vi "AddModule_Item_OnPopupMenu.vi"(11 "Object":T1) -> ()   [LabVIEW 2012]
doc: "OnPopupMenu\n\n\nInputs:\n---------------------\n- Object : U64; \n\nOutputs:\n---------------------\n\n\n----------------------------------------------\n6/8/2018 jcm\nZühlke Engineering AG\nCH-8952 Schlieren\nwww.zuehlke.com"
uses:
  <resource>/Framework/Providers/API/mxLvMenuItem.ctl
  <vilib>/Utility/config.llb/NI_LVConfig.lvlib
  <vilib>/Utility/config.llb/Read Key (String).vi
  <resource>/Framework/Providers/API/ItemRef.ctl
panel:
  out "error out":errorcluster
  in  "error in":errorcluster
  # "Connector Pane"
  # "Locals"
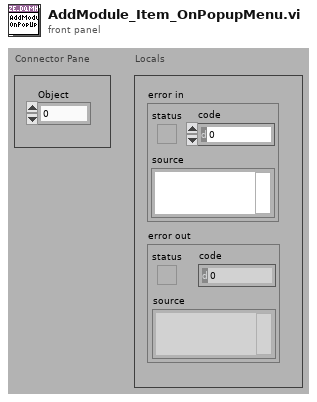
[diagram p1: front panel]
types:
  T1 = typedef "ItemRef.ctl" = u64
  T2 = typedef "mxLvMenuItem.ctl" = cluster{"Menu Name":string, "Description":string, "Icon File Name":path, "Menu Tag":string, "Enabled":bool, "Checked":bool, "Separator":bool, "Batchable":bool, "Weight":i32, "Batch Mode (Ignored if Not Batchable)":enum32{"Show If All Items Support Command", "Show If Any Items Support Command"}, "Menu Location":enum32{"<None>", "Project", "Project / Build Specifications", "Tools", "Tools / Source Control", "Tools / Real-Time Module", "Help"}, "Exclude From Getting Started Window Menu":bool}
  T3 = typedef "NI_LVConfig.lvlib/Config Data RefNum.ctl" = refnum<k1>
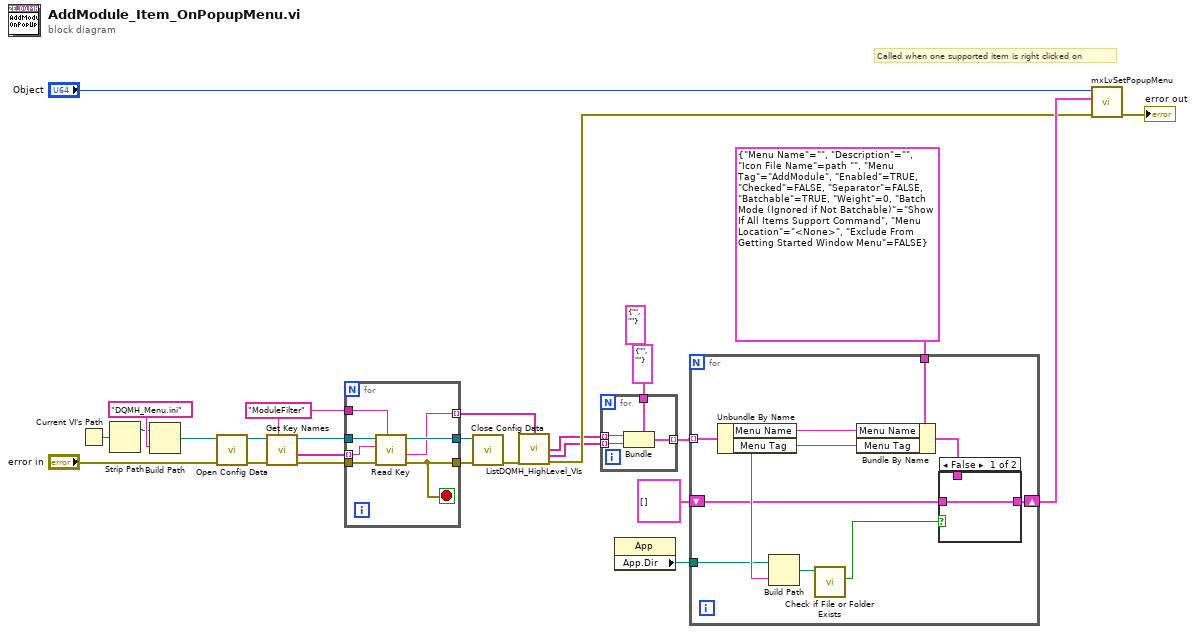
[diagram p0: block diagram]
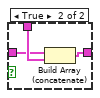
[diagram p2: hidden frame]
diagram:
  (unwired) cluster{"Menu Name":string, "Menu Tag":string} {"Menu Name"="", "Menu Tag"=""}
  w9 = "ModuleFilter" ("section (optional)")
  # "Called when one supported item is right clicked on"
  n1 = Current VI's Path() -> (path=w16:path)
  n2 = Strip Path(path=w16) -> (stripped path=w15:path)  [unwired: 1 out]
  n3 = Build Path(base path=w15, name or relative path="DQMH_Menu.ini") -> (appended path=w18:path)
  n4 = call <vilib>:"Open Config Data.vi"("error in (no error)"="error in", "configuration file path"=w18) -> ("error out"=w19:errorcluster, "refnum"=w20:T3)  [unwired: 7 in, 1 out]
  n5 = call <vilib>:"Get Key Names.vi"("section"=w9, "error in (no error)"=w19, "refnum"=w20) -> ("error out"=w13:errorcluster, "key names"=w12:string[], "refnum out"=w14:T3)  [unwired: 5 in, 1 out]
  n6 = for {
    tunnel: w14 -> [w33]
    tunnel: w13 -> [w32]
    tunnel: w12 -> [w31] mode=indexing
    tunnel: [w30] -> w11
    tunnel: [w29] -> w10
    tunnel: [w28] -> w4 mode=indexing
    tunnel: w9 -> [w27]
    stop <- w29 stop-if-true
    n7 = call-poly <vilib>:"Read Key.vi"("section"=w27, "error in (no error)"=w32, "key"=w31, "refnum"=w33) -> ("error out"=w29:errorcluster, "value"=w28:string, "refnum out"=w30:T3)  [unwired: 4 in, 1 out]
  }
  n8 = call <vilib>:"Close Config Data.vi"("error in (no error)"=w10, "refnum"=w11) -> ("error out"=w6:errorcluster)  [unwired: 8 in, 1 out]
  n9 = call "ListDQMH_HighLevel_VIs.vi"("Filter"=w4, "error in"=w6) -> ("Module_Name"=w2:string[], "Module_Tag"=w1:string[], "error IO"=w5:errorcluster)  [unwired: 9 in, 2 out]
  n10 = for {
    tunnel: cluster{"Menu Name":string, "Menu Tag":string} {"Menu Name"="", "Menu Tag"=""} -> [w37]
    tunnel: [w36] -> w3 mode=indexing
    tunnel: w2 -> [w35] mode=indexing
    tunnel: w1 -> [w34] mode=indexing
    n11 = Bundle(cluster=w37, "Menu Name"=w35, "Menu Tag"=w34) -> (w36:cluster{"Menu Name":string, "Menu Tag":string})
  }
  n12 = property class="App"() -> ("App.Dir"=w24:path)  [unwired: 2 in, 2 out]
  n13 = for {
    tunnel: w3 -> [w46] mode=indexing
    tunnel: T2 {"Menu Name"="", "Description"="", "Icon File Name"=path "", "Menu Tag"="AddModule", "Enabled"=TRUE, "Checked"=FALSE, "Separator"=FALSE, "Batchable"=TRUE, "Weight"=0, "Batch Mode (Ignored if Not Batchable)"=enum."Show If All Items Support Command", "Menu Location"=enum."<None>", "Exclude From Getting Started Window Menu"=FALSE} ("Menu Item") -> [w47]
    tunnel: w24 -> [w43]
    shift-right: [w41] -> w21
    shift-left: T2[] [] -> [w39]
    n14 = Unbundle By Name(w46) -> ("Menu Name"=w45:string, "Menu Tag"=w44:string)
    n15 = Build Path(base path=w43, name or relative path=w44) -> (appended path=w42:path)
    n16 = call <vilib>:"Check if File or Folder Exists.vi"("path"=w42) -> ("file or folder exists?"=w38:bool)  [unwired: 8 in, 2 out]
    n17 = Bundle By Name(cluster=w47, "Menu Name"=w45, "Menu Tag"=w44) -> (w40:T2)
    n18 = case shown="False" w38 {
      tunnel: [w48 w51] -> w41
      tunnel: w40 -> [_ w50]
      tunnel: w39 -> [w48 w49]
      frame False {
      }
      frame True {
        n19 = Build Array (concatenate)(w49, w50) -> (w51:T2[])
      }
    }
  }
  n20 = call <resource>:"mxLvSetPopupMenu.vi"("error in"=w5, "Popup Menu Items"=w21, "Item"="Object") -> ("error out"=→"error out":errorcluster)  [unwired: 7 in, 1 out]
